vi "Conductivity_Calibration_Logger.vi"() -> ()   [LabVIEW 2011]
panel:
  out "Analog Values":dbl[](array[numeric])
  in  "Tab Control":enum32{"Display", "DAQ"}(tab)
  in  "Column Headers":string[](array[string])=["Water Mass (g)", "NaCl Mass (g)", "Board Response Vpk-pk", "Extern Temp °F", "None", "Foxboro Cond", "Foxboro °F", "D 7"]
  in  "Data Entered":string[](array[string])=["1000", "20", "6.153"]
  out "Measurements":string[](array[string])
  in  "External Save Signal":bool
  in  "Save Interval [s]":dbl=99999.0 min=0.0
  in  "Save Enable":bool=TRUE
  out "File Path":path
  out "Save Error":errorcluster
  in  "File Name":string="Cond_Calib"
  in  "Folder Location":path=path "C:/"
  in  "Scale Template":T1={"Channel Select"=0, "Clear/Reset Scales"=FALSE, "Channel #"=["0", "1", "2", "3", "4", "5", "6", "7", "8", "9", "10", "11", "12", "13", "14", "15", "16", "17", "18", "19", "20", "21", "22", "23", "24", "25", "26", "27", "28", "29", "30", "31"], "Scale Names"=["0", "1", "2", "3", "4", "5", "6", "7", "8", "9", "10", "11", "12", "13", "14", "15", "16", "17", "18", "19", "20", "21", "22", "23", "24", "25", "26", "27", "28", "29", "30", "31"], "Set?"=[FALSE, FALSE, FALSE, FALSE, FALSE, FALSE, FALSE, FALSE, FALSE, FALSE, FALSE, FALSE, FALSE, FALSE, FALSE, FALSE, FALSE, FALSE, FALSE, FALSE, FALSE, FALSE, FALSE, FALSE, FALSE, FALSE, FALSE, FALSE, FALSE, FALSE, FALSE, FALSE, FALSE, FALSE, FALSE, FALSE, FALSE, FALSE, FALSE, FALSE, FALSE, FALSE, FALSE, FALSE, FALSE, FALSE, FALSE, FALSE, FALSE, FALSE, FALSE, FALSE, FALSE, FALSE, FALSE, FALSE, FALSE, FALSE, FALSE, FALSE, FALSE, FALSE, FALSE, FALSE], "HI/LO Setpoints"=[1.0, 0.0, 1.0, 0.0, 1.0, 0.0, 1.0, 0.0, 1.0, 0.0, 1.0, 0.0, 1.0, 0.0, 1.0, 0.0, 1.0, 0.0, 1.0, 0.0, 1.0, 0.0, 1.0, 0.0, 1.0, 0.0, 1.0, 0.0, 1.0, 0.0, 1.0, 0.0, 1.0, 0.0, 1.0, 0.0, 1.0, 0.0, 1.0, 0.0, 1.0, 0.0, 1.0, 0.0, 1.0, 0.0, 1.0, 0.0, 1.0, 0.0, 1.0, 0.0, 1.0, 0.0, 1.0, 0.0, 1.0, 0.0, 1.0, 0.0, 1.0, 0.0, 1.0, 0.0], "Units"=["0", "1", "2", "3", "4", "5", "6", "7", "8", "9", "10", "11", "12", "13", "14", "15", "16", "17", "18", "19", "20", "21", "22", "23", "24", "25", "26", "27", "28", "29", "30", "31"], "HI/LO Signals"=[1.0, 0.0, 1.0, 0.0, 1.0, 0.0, 1.0, 0.0, 1.0, 0.0, 1.0, 0.0, 1.0, 0.0, 1.0, 0.0, 1.0, 0.0, 1.0, 0.0, 1.0, 0.0, 1.0, 0.0, 1.0, 0.0, 1.0, 0.0, 1.0, 0.0, 1.0, 0.0, 1.0, 0.0, 1.0, 0.0, 1.0, 0.0, 1.0, 0.0, 1.0, 0.0, 1.0, 0.0, 1.0, 0.0, 1.0, 0.0, 1.0, 0.0, 1.0, 0.0, 1.0, 0.0, 1.0, 0.0, 1.0, 0.0, 1.0, 0.0, 1.0, 0.0, 1.0, 0.0], "Slope/Intercept"=[1.0, 0.0, 1.0, 0.0, 1.0, 0.0, 1.0, 0.0, 1.0, 0.0, 1.0, 0.0, 1.0, 0.0, 1.0, 0.0, 1.0, 0.0, 1.0, 0.0, 1.0, 0.0, 1.0, 0.0, 1.0, 0.0, 1.0, 0.0, 1.0, 0.0, 1.0, 0.0, 1.0, 0.0, 1.0, 0.0, 1.0, 0.0, 1.0, 0.0, 1.0, 0.0, 1.0, 0.0, 1.0, 0.0, 1.0, 0.0, 1.0, 0.0, 1.0, 0.0, 1.0, 0.0, 1.0, 0.0, 1.0, 0.0, 1.0, 0.0, 1.0, 0.0, 1.0, 0.0], "IN/OUT Values"=[0.0, 0.0, 0.0, 0.0, 0.0, 0.0, 0.0, 0.0, 0.0, 0.0, 0.0, 0.0, 0.0, 0.0, 0.0, 0.0, 0.0, 0.0, 0.0, 0.0, 0.0, 0.0, 0.0, 0.0, 0.0, 0.0, 0.0, 0.0, 0.0, 0.0, 0.0, 0.0, 0.0, 0.0, 0.0, 0.0, 0.0, 0.0, 0.0, 0.0, 0.0, 0.0, 0.0, 0.0, 0.0, 0.0, 0.0, 0.0, 0.0, 0.0, 0.0, 0.0, 0.0, 0.0, 0.0, 0.0, 0.0, 0.0, 0.0, 0.0, 0.0, 0.0, 0.0, 0.0], "Sim Signals?"=FALSE, "Sim. Signal"=0.0} {"Sim. Signal" format="%#.3p"; "Channel Select" min=0 step=1; "Slope/Intercept" format="%#.3p"; "HI/LO Setpoints" format="%#.3p"; "IN/OUT Values" format="%#.3p"; "HI/LO Signals" format="%#.3p"}
  in  "9219 Settings":T2={"Sample Rate [Hz]"=50.0, "Number of Samples"=50, "Rolling Average"=2, "AI.ADCTimingMode"=14714} {"AI.ADCTimingMode" items=["High Resolution"=10195, "High Speed"=14712, "Best 50 Hz Rejection"=14713, "Best 60 Hz Rejection"=14714, "Custom"=10137]; "Sample Rate [Hz]" format="%#_6p"}
  out "Scale Error":errorcluster={"status"=FALSE, "code"=1073676294, "source"="VISA Read in ICP Analog Input (SubVI).vi->AquaLogic_Test_Life_Test.vi"}
  in  "Wait (ms)":u32=10
  out "ui":i32=42
  out "daq":i32=155
  out "Analog Error":errorcluster
  in  "9219 Device Name":tag
  in  "STOP PROGRAM":bool=TRUE
  # "Last Updated 4-18-2012"
  # "Ch.\n#"
  # "Scale\nName"
  # "Set\nValues?"
  # "Channel\nSelect"
  # "Scaled"
  # "Pre-Scaled"
  # "Scaling Result"
  # "Values"
  # "Units"
  # "Values"
  # "HI"
  # "Slope"
  # "IN"
  # "LO"
  # "Intercept"
  # "OUT"
  # "HI"
  # "Slope"
  # "IN"
  # "LO"
  # "Intercept"
  # "OUT"
  # "HI"
  # "Slope"
  # "IN"
  # "LO"
  # "Intercept"
  # "OUT"
  # "HI"
  # "Slope"
  # "IN"
  # "LO"
  # "Intercept"
  # "OUT"
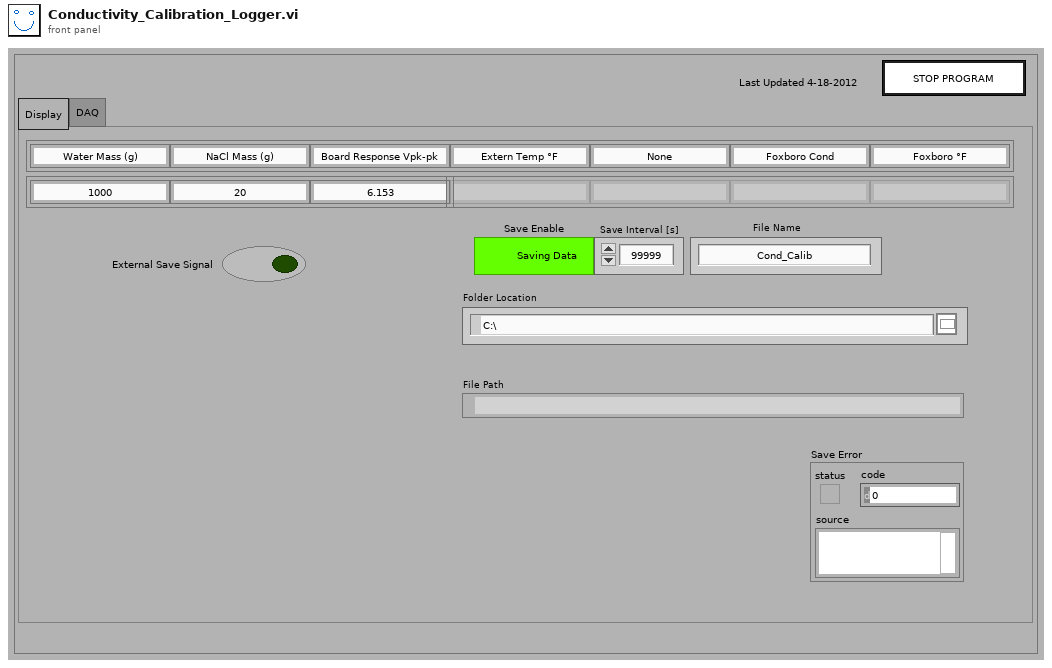
[diagram p1: front panel]
types:
  T1 = cluster{"Channel Select":i32, "Clear/Reset Scales":bool, "Channel #":string[], "Scale Names":string[], "Set?":bool[], "HI/LO Setpoints":dbl[], "Units":string[], "HI/LO Signals":dbl[], "Slope/Intercept":dbl[], "IN/OUT Values":dbl[], "Sim Signals?":bool, "Sim. Signal":dbl}
  T2 = cluster{"Sample Rate [Hz]":dbl, "Number of Samples":i32, "Rolling Average":i32, "AI.ADCTimingMode":i32}
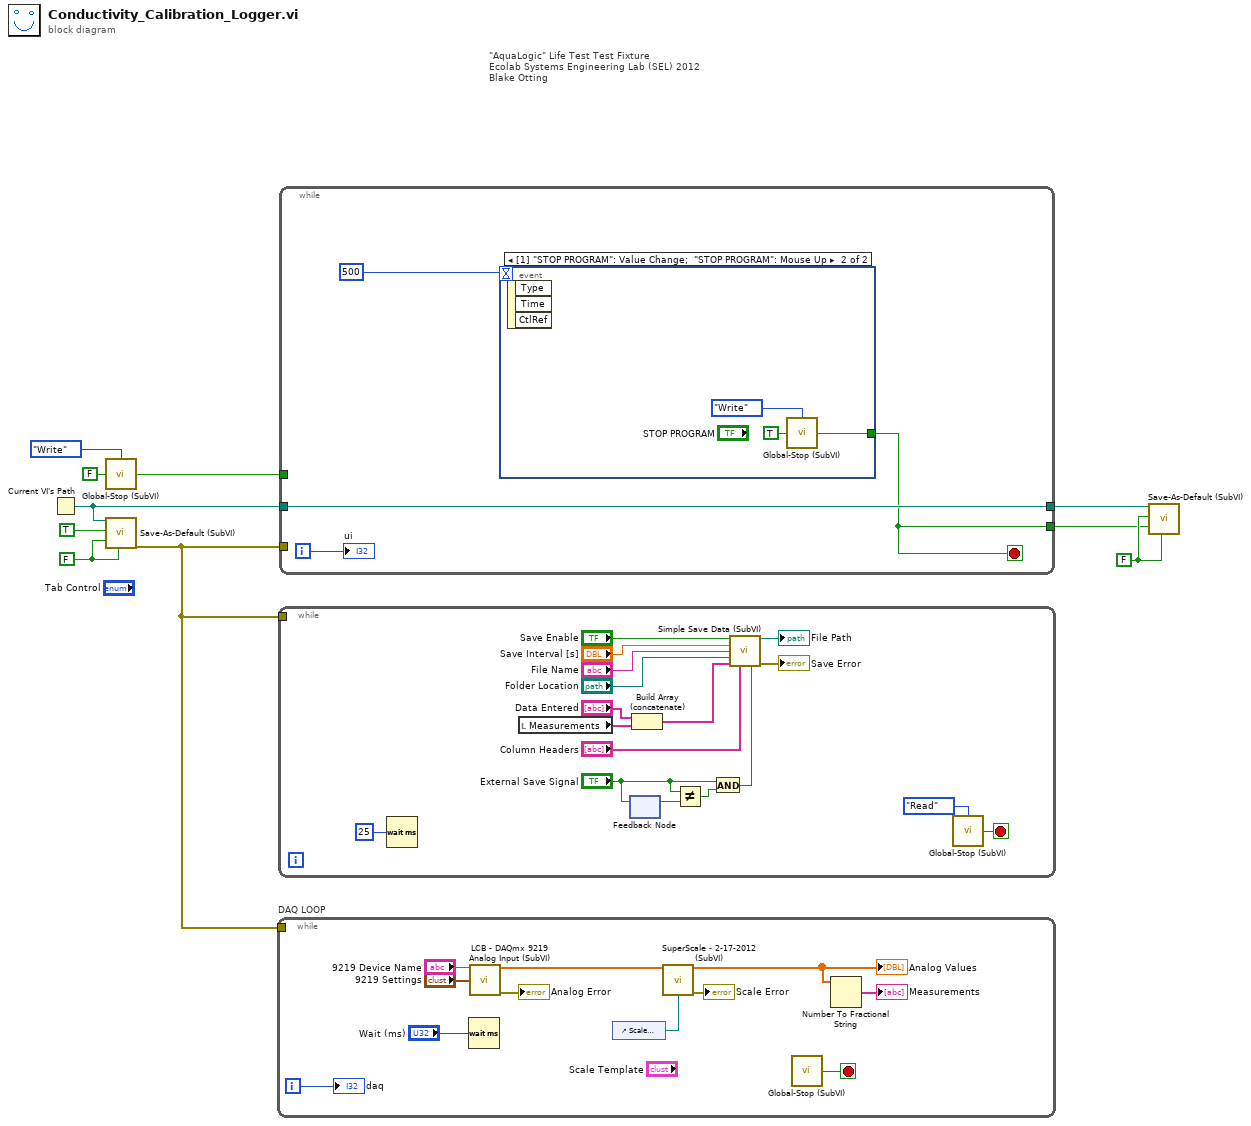
[diagram p0: block diagram]
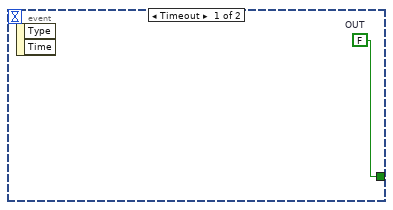
[diagram p2: hidden frame]
diagram:
  w2 = FALSE
  w9 = FALSE
  # "\"AquaLogic\" Life Test Test Fixture\nEcolab Systems Engineering Lab (SEL) 2012\nBlake Otting"
  n1 = Current VI's Path() -> (path=w6:path)
  n2 = call "Global-Stop (SubVI).vi"("Mode (Read)"=enum16{"Read", "Write"}."Write", "IN"=FALSE) -> ("OUT"=w3:bool)  [unwired: 2 in]
  n3 = call "Save-As-Default (SubVI).vi"("Current VI's Path"=w6, "Load Settings"=TRUE, "Save Settings"=w2, "Save and Exit"=w2) -> ("Save as Default Error"=w1:errorcluster)  [unwired: 15 in]
  n4 = while "DAQ LOOP" {
    tunnel: w1 -> [_]
    i -> [w20]
    stop <- w21 stop-if-true
    n5 = Wait (ms)(milliseconds to wait="Wait (ms)") -> ()  [unwired: 1 out]
    n6 = call "LCB - DAQmx 9219 Analog Input (SubVI).vi"("9219 Device Name"="9219 Device Name", "9219 Settings"="9219 Settings") -> ("9219 Signals"=w16:dbl[], "Analog Error"=→"Analog Error":errorcluster)  [unwired: 12 in]
    n7 = control-ref of="Scale Template"() -> (w17:refnum<vi>)
    n8 = call "SuperScale - 2-17-2012 (SubVI).vi"("Measured Signals"=w16, "Scale Reference"=w17) -> ("Scaled Values"=w13:dbl[], "Scale Error"=→"Scale Error":errorcluster)  [unwired: 12 in]
    "Analog Values" <- w13
    n9 = call "Global-Stop (SubVI).vi"() -> ("OUT"=w21:bool)  [unwired: 4 in]
    n10 = Number To Fractional String(number=w13) -> (F-format string=→"Measurements":string[])  [unwired: 3 in]
    "daq" <- w20
  }
  n11 = while {
    tunnel: w1 -> [_]
    stop <- w37 stop-if-true
    n12 = Wait (ms)(milliseconds to wait=u32 25) -> ()  [unwired: 1 out]
    n13 = local read "Measurements"() -> (w28:string[])
    n14 = feedback-in #1("External Save Signal") -> ()
    n15 = feedback #1() -> (w25:bool)  [unwired: 1 in]
    n16 = Build Array (concatenate)("Data Entered", w28) -> (w27:string[])
    n17 = Not Equal?(x="External Save Signal", y=w25) -> (x != y?=w23:bool)
    n18 = And(x="External Save Signal", y=w23) -> (x .and. y?=w22:bool)
    n19 = call "Simple Save Data (SubVI).vi"("Save Enable"="Save Enable", "Save Interval [s]"="Save Interval [s]", "File Name"="File Name", "Folder Location"="Folder Location", "Data Array (Row)"=w27, "Column Header Array"="Column Headers", "External Save Signal"=w22) -> ("File Path"=→"File Path":path, "Save Error"=→"Save Error":errorcluster)  [unwired: 6 in, 1 out]
    n20 = call "Global-Stop (SubVI).vi"("Mode (Read)"=enum16{"Read", "Write"}."Read") -> ("OUT"=w37:bool)  [unwired: 3 in]
  }
  n21 = while {
    tunnel: [w39] -> w8
    tunnel: [w42] -> w7
    tunnel: w6 -> [w42]
    tunnel: w3 -> [_]
    tunnel: w1 -> [_]
    i -> [w41]
    stop <- w39 stop-if-true
    n22 = event shown="[1] \"STOP PROGRAM\": Value Change;  \"STOP PROGRAM\": Mouse Up" {
      selector: _ -> [_ _]
      dyn-events: _ -> [_ _]
      timeout: 500 -> [_ _]
      tunnel: [w43 w44] -> w39
      event Timeout {
        w43 = FALSE  # OUT
        n23 = event-data() -> ()  [unwired: 1 in, 2 out]
      }
      event "STOP PROGRAM": Value Change; "STOP PROGRAM": Mouse Up {
        n24 = event-data() -> ()  [unwired: 1 in, 3 out]
        n25 = call "Global-Stop (SubVI).vi"("Mode (Read)"=enum16{"Read", "Write"}."Write", "IN"=TRUE) -> ("OUT"=w44:bool)  [unwired: 2 in]
      }
    }
    "ui" <- w41
  }
  n26 = call "Save-As-Default (SubVI).vi"("Current VI's Path"=w7, "Load Settings"=w9, "Save Settings"=w8, "Save and Exit"=w9) -> ()  [unwired: 15 in, 1 out]
